vi "Periodic Tasks.vi"(8 "error in":errorcluster) -> ()   [LabVIEW 2013]
doc: "This VI runs in parallel to other tasks. It can contain as many user-defined periodic loops as you need. These can carry out PID or other sorts of timed response."
uses:
  <vilib>/Rock Robotics/WPI/DriverStation/DriverStationLCD/WPI_DriverStationLCDLCDLine.ctl
  <vilib>/Rock Robotics/SystemInterfaces/Utilities/FPGA_UtilitiesLED Source.ctl
  <vilib>/Rock Robotics/SystemInterfaces/Utilities/FPGA_UtilitiesLED State.ctl
  <vilib>/Rock Robotics/WPI/Relay/WPI_RelayValue.ctl
  <vilib>/Rock Robotics/WPI/SafetyOutput/WPI_SafetyOutputConfigMenu.ctl
  <vilib>/Rock Robotics/WPI/DriverStation/WPI_DriverStationRobotMode2.ctl
  <vilib>/Rock Robotics/WPI/Solenoid/WPI_SolenoidValue.ctl
  Begin/Global Refnums.vi
  <vilib>/Rock Robotics/WPI/Solenoid/WPI_SolenoidSetEnum.vi
  Begin/Robot Global Data.vi
  Begin/Global Variables.vi
  <vilib>/Rock Robotics/WPI/Joystick/WPI_JoystickGetSetRefNum.vi
  <vilib>/Rock Robotics/WPI/Compressor/WPI_CompressorGetSetRefNum.vi
panel:
  out "Fire":bool
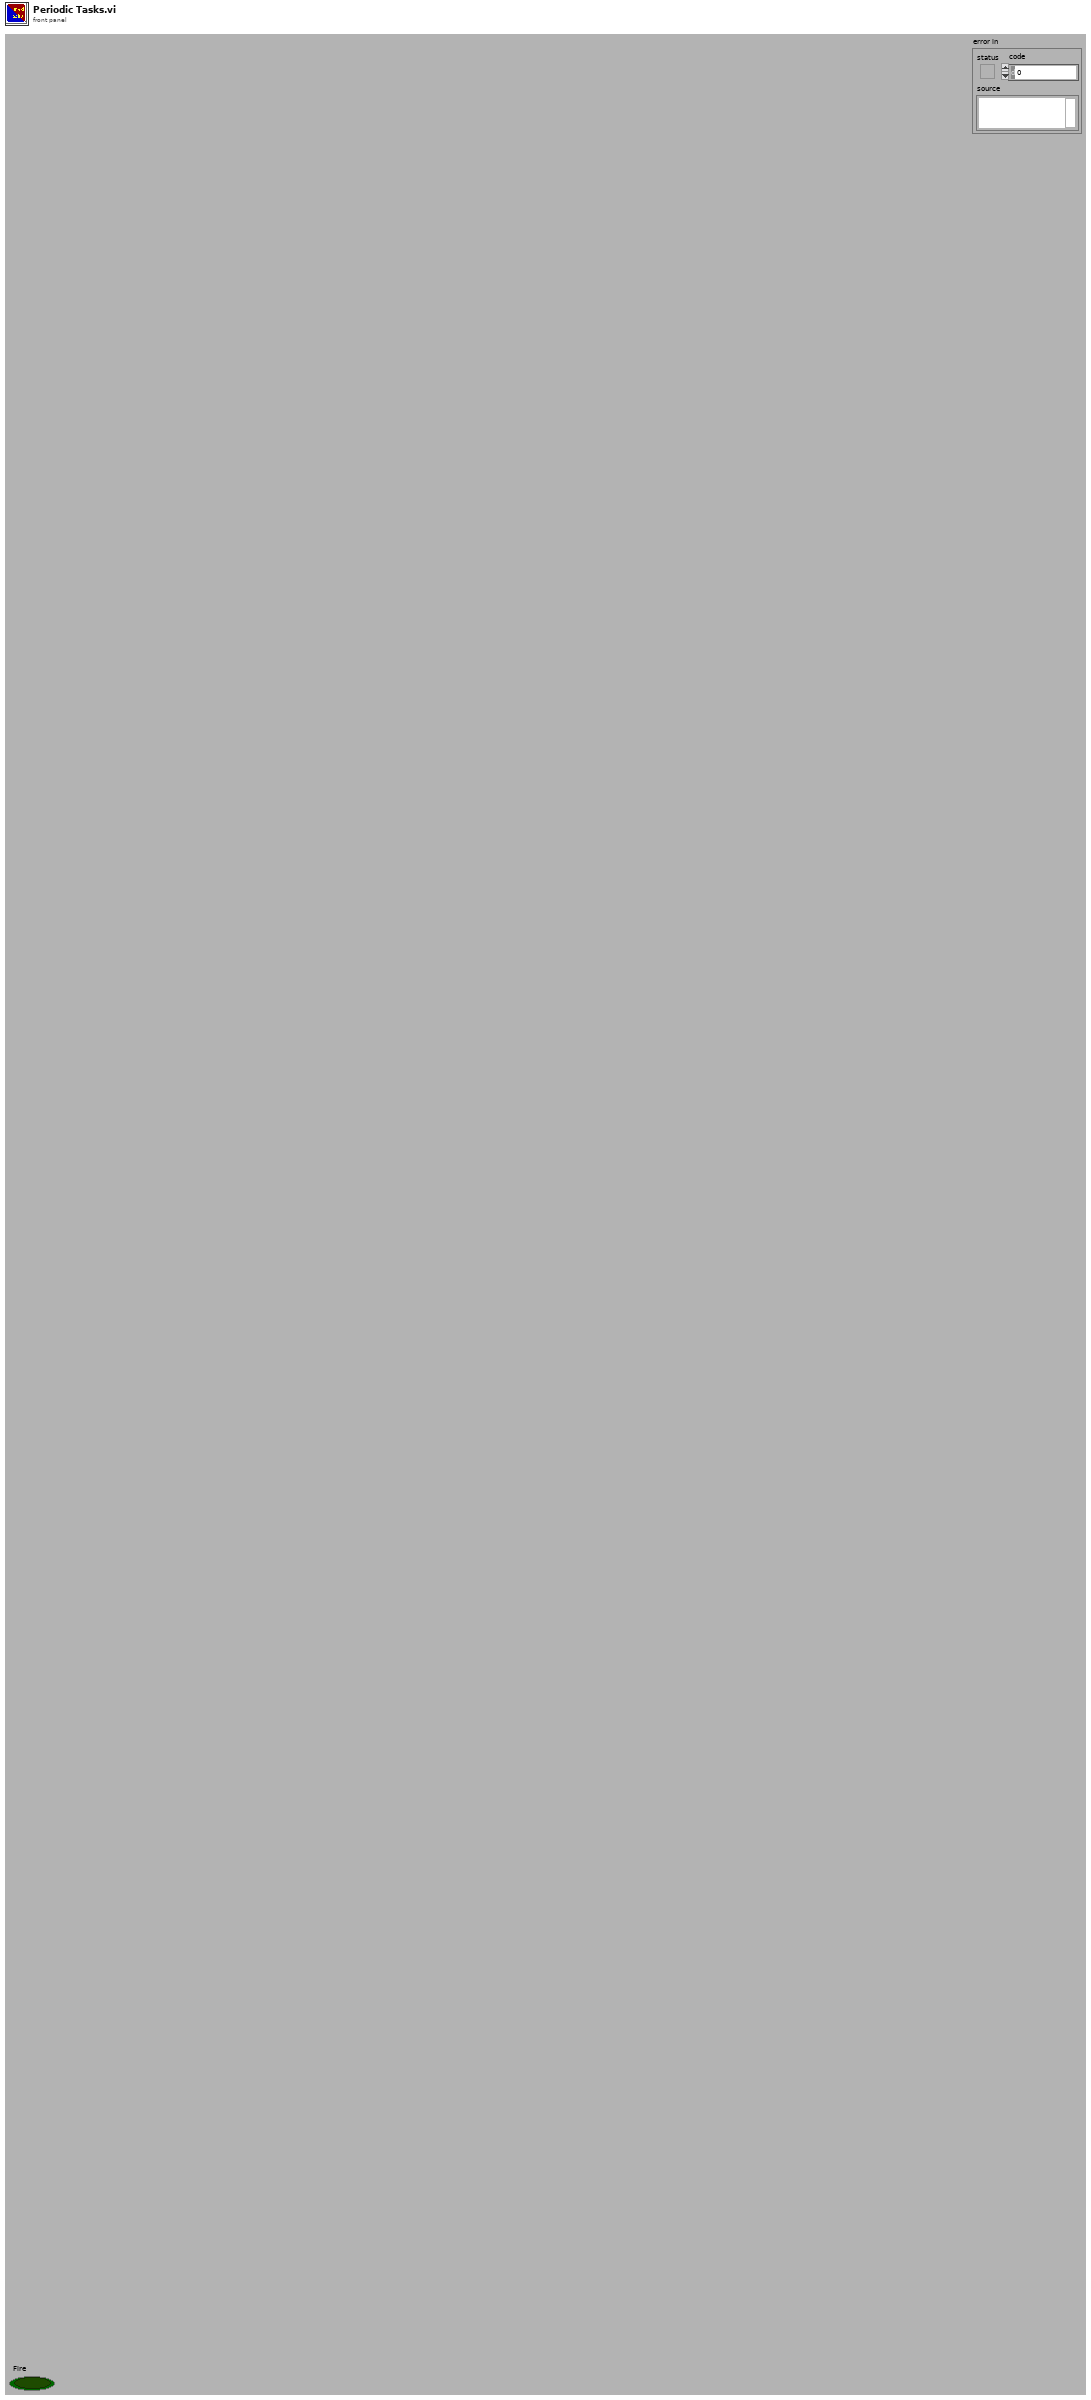
[diagram p1: front panel]
types:
  T1 = typedef "WPI_DriverStationLCDLCDLine.ctl" = enum16{"Main - Line 1", "User - Line 2", "User - Line 3", "User - Line 4", "User - Line 5", "User - Line 6"}
  T2 = typedef "WPI_SolenoidValue.ctl" = enum16{"Off", "On", "Forward", "Reverse"}
  T3 = typedef "WPI_SafetyOutputConfigMenu.ctl" = enum16{"Enable", "Disable"}
  T4 = typedef "WPI_SolenoidDevRef.ctl" = cluster{"DevStatus":errorcluster, "Solenoid Module":T5, "Forward Solenoid Channel":T6, "Reverse Solenoid Channel":T6}
  T5 = typedef "FPGA_TypedefSolenoidModule.ctl" = enum16{"Solenoid Module 1", "Solenoid Module 2"}
  T6 = typedef "WPI_SolenoidChannel.ctl" = enum8{"Solenoid 1", "Solenoid 2", "Solenoid 3", "Solenoid 4", "Solenoid 5", "Solenoid 6", "Solenoid 7", "Solenoid 8", "Invalid"}
  T7 = typedef "WPI_RelayValue.ctl" = enum16{"Off", "On", "Forward", "Reverse"}
  T8 = typedef "WPI_CompressorDevRef.ctl" = cluster{"DevStatus":errorcluster, "DigitalInputDevRef":T9, "RelayDevRef":T12}
  T9 = typedef "WPI_DigitalInputDevRef.ctl" = cluster{"DevStatus":errorcluster, "DIO Channel":T10, "Digital Module":T11}
  T10 = typedef "FPGA_DIOChannel.ctl" = enum8{"DIO 1", "DIO 2", "DIO 3", "DIO 4", "DIO 5", "DIO 6", "DIO 7", "DIO 8", "DIO 9", "DIO 10", "DIO 11", "DIO 12", "DIO 13", "DIO 14", "Invalid"}
  T11 = typedef "FPGA_TypedefDigitalModule.ctl" = enum16{"Digital Module 1", "Digital Module 2"}
  T12 = typedef "WPI_RelayDevRef.ctl" = cluster{"DevStatus":errorcluster, "Relay Channel":T13, "Digital Module":T11, "Relay Direction":T14}
  T13 = typedef "FPGA_DIORelayChannel.ctl" = enum8{"Relay 1", "Relay 2", "Relay 3", "Relay 4", "Relay 5", "Relay 6", "Relay 7", "Relay 8", "Invalid"}
  T14 = typedef "WPI_RelayDirection.ctl" = enum16{"Both directions", "Forward only", "Reverse only"}
  T15 = typedef "WPI_EncoderDevRef.ctl" = cluster{"DevStatus":errorcluster, "EncoderIndex":T16, "CounterIndex":T17, "DistancePerCount":dbl, "Decoding Type":T18}
  T16 = typedef "FPGA_EncoderIdx.ctl" = enum8{"Enc 0", "Enc 1", "Enc 2", "Enc 3", "Invalid"}
  T17 = typedef "FPGA_CounterCtrSystemIndex.ctl" = enum8{"Ctr 0", "Ctr 1", "Ctr 2", "Ctr 3", "Ctr 4", "Ctr 5", "Ctr 6", "Ctr 7", "Invalid"}
  T18 = typedef "WPI_EncoderType.ctl" = enum16{"1x", "2x", "4x"}
  T19 = typedef "WPI_DriverStationRobotMode2.ctl" = enum16{"Autonomous Disabled", "Autonomous Enabled", "Teleop Disabled", "Teleop Enabled", "Timeout", "Finish", "Test Disabled", "Test Enabled"}
  T20 = typedef "WPI_JoystickDevRef.ctl" = cluster{"Device":T21}
  T21 = typedef "WPI_JoystickDeviceEnum.ctl" = enum16{"USB 1", "USB 2", "USB 3", "USB 4", "Kinect 1", "Kinect 2"}
  T22 = typedef "WPI_JoystickButtonState.ctl" = cluster{"Button 1":bool, "Button 2":bool, "Button 3":bool, "Button 4":bool, "Button 5":bool, "Button 6":bool, "Button 7":bool, "Button 8":bool, "Button 9":bool, "Button 10":bool, "Button 11":bool, "Button 12":bool}
  T23 = typedef "WPI_MotorControlDeviceRef.ctl" = cluster{"DeviceStatus":errorcluster, "Type":enum16{"PWM", "CAN"}, "PWM":cluster{"Digital Module":T11, "PWM Channel":T24, "DeadBand":T25}, "CAN":cluster{"Device Number":u8, "Control Mode":T26, "Semaphore":T27, "Max Vout":dbl}, "Invert":bool, "TransformRef":T28, "InvTransformRef":T28}
  T24 = typedef "FPGA_DIOPWMChannel.ctl" = enum8{"PWM 1", "PWM 2", "PWM 3", "PWM 4", "PWM 5", "PWM 6", "PWM 7", "PWM 8", "PWM 9", "PWM 10", "Invalid"}
  T25 = typedef "WPI_PWMDeadband.ctl" = cluster{"Name":string, "maxPositivePwm":i32, "minPositivePwm":i32, "centerPwm":i32, "maxNegativePwm":i32, "minNegativePwm":i32, "angularRange":u16}
  T26 = typedef "WPI_CANJaguar_ControlMode.ctl" = enum8{"Percent VBus", "Current", "Speed", "Position", "Voltage"}
  T27 = typedef "Semaphore RefNum" = refnum<k1>
  T28 = typedef "WPI_PWMTransform_ConPane.ctl" = refnum<vi>
  T29 = typedef "FPGA_UtilitiesLED State.ctl" = enum16{"Off", "On", "Toggle"}
  T30 = typedef "FPGA_UtilitiesLED Source.ctl" = enum16{"User LED", "FPGA LED"}
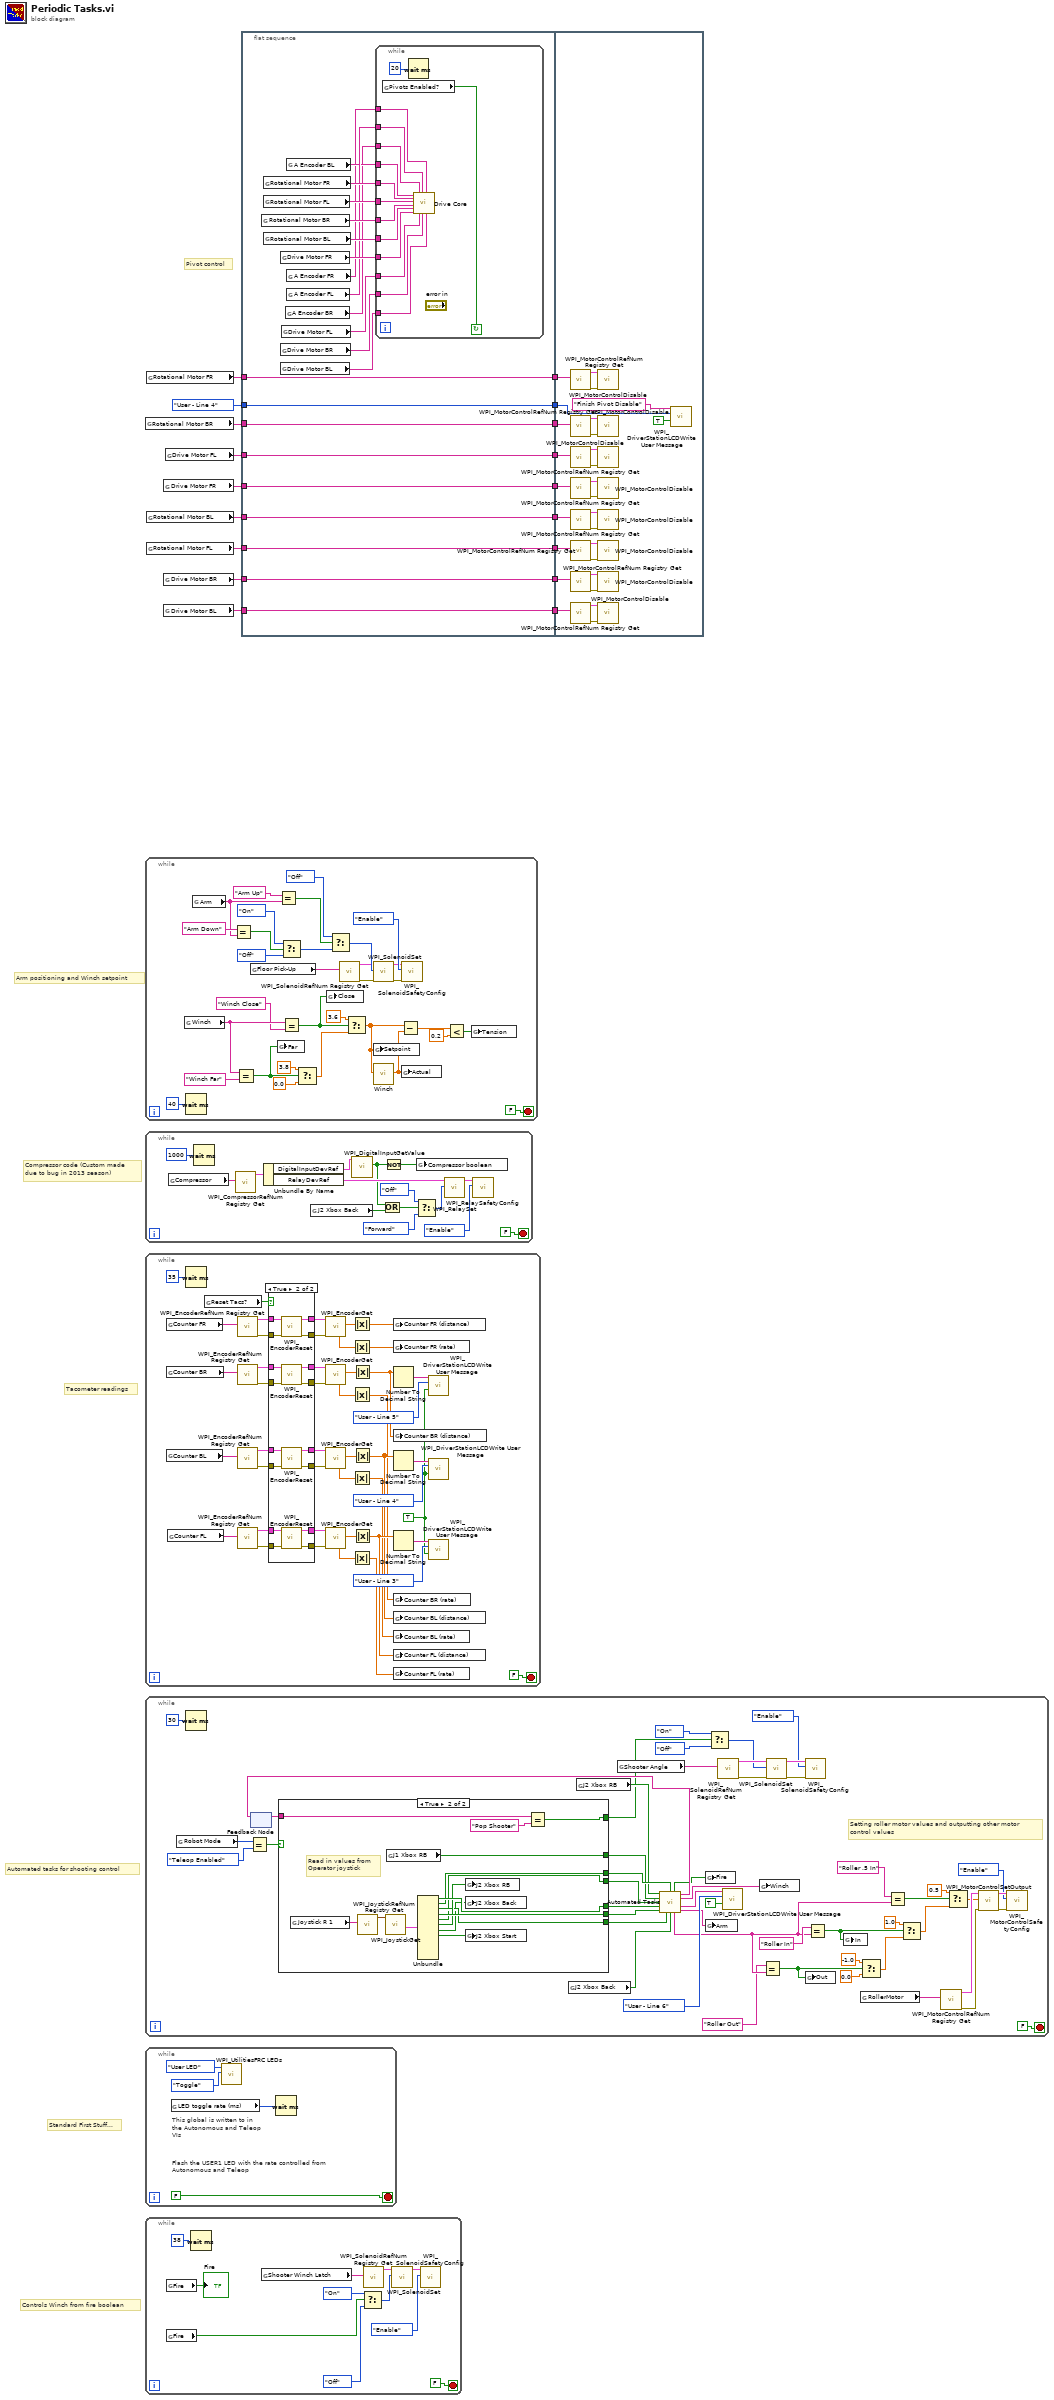
[diagram p0: block diagram]
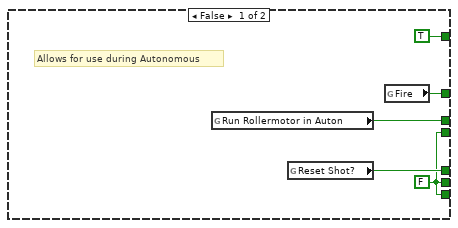
[diagram p2: hidden frame]
diagram:
  # "Automated tasks for shooting control"
  # "Tacometer readings"
  # "Compressor code (Custom made\ndue to bug in 2013 season)"
  # "Arm positioning and Winch setpoint"
  # "Pivot control"
  # "Standard First Stuff..."
  # "Controls Winch from fire boolean"
  n1 = global read "Global Refnums.vi" "Rotational Motor BR"() -> (w16:string)
  n2 = while {
    stop <- FALSE stop-if-true
    n3 = global read "Global Refnums.vi" "Winch"() -> (w50:string)
    n4 = Wait (ms)(milliseconds to wait=u32 40) -> ()  [unwired: 1 out]
    n5 = global read "Global Refnums.vi" "Arm"() -> (w24:string)
    n6 = Equal?(x="Arm Down", y=w24) -> (x = y?=w28:bool)
    n7 = Equal?(x=w50, y="Winch Far") -> (x = y?=w21:bool)
    n8 = global read "Global Refnums.vi" "Floor Pick-Up"() -> (w39:string)
    n9 = global write "Global Refnums.vi" "Far"(w21) -> ()
    n10 = Equal?(x="Arm Up", y=w24) -> (x = y?=w41:bool)
    n11 = Select(t=WPI_SolenoidValue."On" ("Value"), s=w28, f=WPI_SolenoidValue."Off" ("Value")) -> (s? t:f=w27:T2)
    n12 = Equal?(x=w50, y="Winch Close") -> (x = y?=w20:bool)
    n13 = Select(t=3.8, s=w21, f=0.0) -> (s? t:f=w47:dbl)
    n14 = global write "Global Refnums.vi" "Close"(w20) -> ()
    n15 = Select(t=WPI_SolenoidValue."Off" ("Value"), s=w41, f=w27) -> (s? t:f=w43:T2)
    n16 = call <vilib>:"WPI_SolenoidRefNum Registry Get.vi"("refnum name"=w39) -> ("error out"=w34:errorcluster, "SolenoidDevRef"=w35:T4)  [unwired: 9 in]
    n17 = Select(t=3.6, s=w20, f=w47) -> (s? t:f=w19:dbl)
    n18 = call-poly <vilib>:"WPI_SolenoidSet.vi"("error in (no error)"=w34, "Value"=w43, "SolenoidDevRef"=w35) -> ("error out"=w37:errorcluster, "SolenoidDevRef"=w36:T4)  [unwired: 7 in]
    n19 = global write "Global Refnums.vi" "Setpoint"(w19) -> ()
    n20 = call "Winch.vi"("setpoint"=w19) -> ("Actual"=w22:dbl)  [unwired: 10 in]
    n21 = Subtract(x=w19, y=w22) -> (x-y=w31:dbl)
    n22 = call <vilib>:"WPI_SolenoidSafetyConfig.vi"("error in (no error)"=w37, "mode"=WPI_SafetyOutputConfigMenu."Enable", "SolenoidDevRef"=w36) -> ()  [unwired: 7 in, 2 out]
    n23 = global write "Global Refnums.vi" "Actual"(w22) -> ()
    n24 = Less?(x=w31, y=0.2) -> (x < y?=w23:bool)
    n25 = global write "Global Refnums.vi" "Tension"(w23) -> ()
  }
  n26 = while {
    stop <- FALSE stop-if-true
    n27 = global read "Global Refnums.vi" "Compressor"() -> (w63:string)
    n28 = Wait (ms)(milliseconds to wait=1000) -> ()  [unwired: 1 out]
    n29 = call <vilib>:"WPI_CompressorRefNum Registry Get.vi"("refnum name"=w63) -> ("CompressorDevRef"=w62:T8)  [unwired: 9 in, 1 out]
    n30 = Unbundle By Name(w62) -> ("DigitalInputDevRef"=w55:T9, "RelayDevRef"=w61:T12)
    n31 = global read "Global Variables.vi" "J2 Xbox Back"() -> (w53:bool)
    n32 = call <vilib>:"WPI_DigitalInputGetValue.vi"("DigitalInputDevRef"=w55) -> ("Value"=w52:bool)  [unwired: 8 in, 2 out]
    n33 = Or(x=w52, y=w53) -> (x .or. y?=w54:bool)
    n34 = Not(x=w52) -> (.not. x?=w51:bool)
    n35 = Select(t=WPI_RelayValue."Off" ("RelayValue"), s=w54, f=WPI_RelayValue."Forward" ("RelayValue")) -> (s? t:f=w58:T7)
    n36 = global write "Global Refnums.vi" "Compressor boolean"(w51) -> ()
    n37 = call <vilib>:"WPI_RelaySet.vi"("RelayValue"=w58, "RelayDevRef"=w61) -> ("RelayDevRef"=w60:T12)  [unwired: 8 in, 1 out]
    n38 = call <vilib>:"WPI_RelaySafetyConfig.vi"("mode"=WPI_SafetyOutputConfigMenu."Enable", "RelayDevRef"=w60) -> ()  [unwired: 8 in, 2 out]
  }
  n39 = while {
    stop <- FALSE stop-if-true
    w67 = TRUE ("clear line before write (T)")
    n40 = global read "Global Refnums.vi" "Counter FR"() -> (w78:string)
    n41 = global read "Global Refnums.vi" "Counter BR"() -> (w76:string)
    n42 = global read "Global Refnums.vi" "Counter BL"() -> (w79:string)
    n43 = global read "Global Refnums.vi" "Counter FL"() -> (w77:string)
    n44 = Wait (ms)(milliseconds to wait=u32 35) -> ()  [unwired: 1 out]
    n45 = global read "Global Variables.vi" "Reset Tacs?"() -> (w66:bool)
    n46 = call <vilib>:"WPI_EncoderRefNum Registry Get.vi"("refnum name"=w78) -> ("error out"=w94:errorcluster, "EncoderDevRef"=w97:T15)  [unwired: 9 in]
    n47 = call <vilib>:"WPI_EncoderRefNum Registry Get.vi"("refnum name"=w76) -> ("error out"=w102:errorcluster, "EncoderDevRef"=w103:T15)  [unwired: 9 in]
    n48 = call <vilib>:"WPI_EncoderRefNum Registry Get.vi"("refnum name"=w79) -> ("error out"=w104:errorcluster, "EncoderDevRef"=w105:T15)  [unwired: 9 in]
    n49 = call <vilib>:"WPI_EncoderRefNum Registry Get.vi"("refnum name"=w77) -> ("error out"=w99:errorcluster, "EncoderDevRef"=w100:T15)  [unwired: 9 in]
    n50 = case shown="True" w66 {
      tunnel: w103 -> [w116 w135]
      tunnel: [w116 w134] -> w108
      tunnel: [w118 w133] -> w109
      tunnel: w102 -> [w118 w132]
      tunnel: [w117 w131] -> w107
      tunnel: [w119 w130] -> w106
      tunnel: w105 -> [w117 w129]
      tunnel: w104 -> [w119 w128]
      tunnel: [w115 w120] -> w101
      tunnel: w100 -> [w115 w127]
      tunnel: w99 -> [w114 w126]
      tunnel: [w114 w121] -> w98
      tunnel: w97 -> [w113 w125]
      tunnel: [w113 w122] -> w96
      tunnel: [w112 w123] -> w95
      tunnel: w94 -> [w112 w124]
      frame False {
      }
      frame True {
        n51 = call <vilib>:"WPI_EncoderReset.vi"("error in (no error)"=w124, "EncoderDevRef"=w125) -> ("error out"=w123:errorcluster, "EncoderDevRef"=w122:T15)  [unwired: 8 in]
        n52 = call <vilib>:"WPI_EncoderReset.vi"("error in (no error)"=w132, "EncoderDevRef"=w135) -> ("error out"=w133:errorcluster, "EncoderDevRef"=w134:T15)  [unwired: 8 in]
        n53 = call <vilib>:"WPI_EncoderReset.vi"("error in (no error)"=w128, "EncoderDevRef"=w129) -> ("error out"=w130:errorcluster, "EncoderDevRef"=w131:T15)  [unwired: 8 in]
        n54 = call <vilib>:"WPI_EncoderReset.vi"("error in (no error)"=w126, "EncoderDevRef"=w127) -> ("error out"=w121:errorcluster, "EncoderDevRef"=w120:T15)  [unwired: 8 in]
      }
    }
    n55 = call <vilib>:"WPI_EncoderGet.vi"("error in (no error)"=w95, "EncoderDevRef"=w96) -> ("Distance"=w91:dbl, "Rate"=w87:dbl)  [unwired: 4 in, 4 out]
    n56 = call <vilib>:"WPI_EncoderGet.vi"("error in (no error)"=w109, "EncoderDevRef"=w108) -> ("Distance"=w90:dbl, "Rate"=w86:dbl)  [unwired: 4 in, 4 out]
    n57 = call <vilib>:"WPI_EncoderGet.vi"("error in (no error)"=w106, "EncoderDevRef"=w107) -> ("Distance"=w92:dbl, "Rate"=w88:dbl)  [unwired: 4 in, 4 out]
    n58 = call <vilib>:"WPI_EncoderGet.vi"("error in (no error)"=w98, "EncoderDevRef"=w101) -> ("Distance"=w93:dbl, "Rate"=w89:dbl)  [unwired: 4 in, 4 out]
    n59 = Absolute Value(x=w91) -> (abs(x)=w75:dbl)
    n60 = Absolute Value(x=w87) -> (abs(x)=w74:dbl)
    n61 = Absolute Value(x=w86) -> (abs(x)=w68:dbl)
    n62 = Absolute Value(x=w88) -> (abs(x)=w70:dbl)
    n63 = Absolute Value(x=w89) -> (abs(x)=w72:dbl)
    n64 = Absolute Value(x=w90) -> (abs(x)=w69:dbl)
    n65 = Absolute Value(x=w92) -> (abs(x)=w71:dbl)
    n66 = Absolute Value(x=w93) -> (abs(x)=w73:dbl)
    n67 = global write "Global Refnums.vi" "Counter FR (distance)"(w75) -> ()
    n68 = global write "Global Refnums.vi" "Counter FR (rate)"(w74) -> ()
    n69 = Number To Decimal String(number=w69) -> (decimal integer string=w85:string)  [unwired: 1 in]
    n70 = global write "Global Refnums.vi" "Counter BR (distance)"(w69) -> ()
    n71 = Number To Decimal String(number=w71) -> (decimal integer string=w83:string)  [unwired: 1 in]
    n72 = Number To Decimal String(number=w73) -> (decimal integer string=w84:string)  [unwired: 1 in]
    n73 = global write "Global Refnums.vi" "Counter BR (rate)"(w68) -> ()
    n74 = global write "Global Refnums.vi" "Counter BL (distance)"(w71) -> ()
    n75 = global write "Global Refnums.vi" "Counter BL (rate)"(w70) -> ()
    n76 = global write "Global Refnums.vi" "Counter FL (distance)"(w73) -> ()
    n77 = global write "Global Refnums.vi" "Counter FL (rate)"(w72) -> ()
    n78 = call <vilib>:"WPI_DriverStationLCDWrite User Message.vi"("line text"=w85, "line"=WPI_DriverStationLCDLCDLine."User - Line 5", "clear line before write (T)"=w67) -> ()  [unwired: 12 in, 1 out]
    n79 = call <vilib>:"WPI_DriverStationLCDWrite User Message.vi"("line text"=w83, "line"=WPI_DriverStationLCDLCDLine."User - Line 4", "clear line before write (T)"=w67) -> ()  [unwired: 12 in, 1 out]
    n80 = call <vilib>:"WPI_DriverStationLCDWrite User Message.vi"("line text"=w84, "line"=WPI_DriverStationLCDLCDLine."User - Line 3", "clear line before write (T)"=w67) -> ()  [unwired: 12 in, 1 out]
  }
  n81 = while {
    stop <- FALSE stop-if-true
    # "Setting roller motor values and outputting other motor\ncontrol values"
    n82 = global read "Robot Global Data.vi" "Robot Mode"() -> (w157:T19)
    n83 = Wait (ms)(milliseconds to wait=u32 30) -> ()  [unwired: 1 out]
    n84 = Equal?(x=w157, y=WPI_DriverStationRobotMode2."Teleop Enabled") -> (x = y?=w158:bool)
    n85 = feedback #1() -> (w153:string)  [unwired: 1 in]
    n86 = case shown="True" w158 {
      tunnel: [w188 w203] -> w141
      tunnel: [w190 w202] -> w169
      tunnel: [w187 w201] -> w168
      tunnel: [w191 w200] -> w167
      tunnel: w153 -> [_ w198]
      tunnel: [TRUE w197] -> w152
      tunnel: [w187 w195] -> w150
      tunnel: [w187 w194] -> w142
      frame False {
        w187 = FALSE ("J1 Xbox RB")
        # "Allows for use during Autonomous"
        n87 = global read "Global Refnums.vi" "Run Rollermotor in Auton"() -> (w190:bool)
        n88 = global read "Global Refnums.vi" "Reset Shot?"() -> (w188:bool)
        n89 = global read "Global Refnums.vi" "Fire"() -> (w191:bool)
      }
      frame True {
        # "Read in values from \nOperator joystick"
        n90 = global read "Global Refnums.vi" "Joystick R 1"() -> (w204:string)
        n91 = call <vilib>:"WPI_JoystickRefNum Registry Get.vi"("refnum name"=w204) -> ("JoystickDevRef"=w206:T20)  [unwired: 9 in, 1 out]
        n92 = call <vilib>:"WPI_JoystickGet.vi"("JoystickDevRef"=w206) -> ("Buttons"=w205:T22)  [unwired: 4 in, 2 out]
        n93 = global read "Global Variables.vi" "J1 Xbox RB"() -> (w200:bool)
        n94 = Unbundle(w205) -> ("Button 1"=w203:bool, "Button 2"=w202:bool, "Button 3"=w195:bool, "Button 4"=w201:bool, "Button 5"=w194:bool, "Button 6"=w196:bool, "Button 7"=w193:bool, "Button 8"=w192:bool)  [unwired: 4 out]
        n95 = global write "Global Variables.vi" "J2 Xbox RB"(w196) -> ()
        n96 = global write "Global Variables.vi" "J2 Xbox Back"(w193) -> ()
        n97 = global write "Global Variables.vi" "J2 Xbox Start"(w192) -> ()
        n98 = Equal?(x=w198, y="Pop Shooter") -> (x = y?=w197:bool)
      }
    }
    n99 = global read "Global Variables.vi" "J2 Xbox Back"() -> (w138:bool)
    n100 = global read "Global Variables.vi" "J2 Xbox RB"() -> (w155:bool)
    n101 = global read "Global Refnums.vi" "Shooter Angle"() -> (w165:string)
    n102 = call "Automated Tasks.vi"("RB"=w155, "B"=w169, "Fire"=w167, "LB"=w142, "A"=w141, "Y"=w168, "X"=w150, "Back"=w138) -> ("Fire"=w151:bool, "Shooter"=w154:string, "Winch"=w140:string, "Case"=w163:string, "Roller"=w147:string, "Arm"=w160:string)  [unwired: 2 in]
    n103 = feedback-in #1(w154) -> ()
    n104 = global write "Global Refnums.vi" "Fire"(w151) -> ()
    n105 = global write "Global Refnums.vi" "Arm"(w160) -> ()
    n106 = Select(t=WPI_SolenoidValue."On" ("Value"), s=w152, f=WPI_SolenoidValue."Off" ("Value")) -> (s? t:f=w170:T2)
    n107 = call <vilib>:"WPI_SolenoidRefNum Registry Get.vi"("refnum name"=w165) -> ("error out"=w177:errorcluster, "SolenoidDevRef"=w176:T4)  [unwired: 9 in]
    n108 = call <vilib>:"WPI_DriverStationLCDWrite User Message.vi"("line text"=w163, "line"=WPI_DriverStationLCDLCDLine."User - Line 6", "clear line before write (T)"=TRUE) -> ()  [unwired: 12 in, 1 out]
    n109 = global write "Global Refnums.vi" "Winch"(w140) -> ()
    n110 = Equal?(x="Roller Out", y=w147) -> (x = y?=w136:bool)
    n111 = call-poly <vilib>:"WPI_SolenoidSet.vi"("error in (no error)"=w177, "Value"=w170, "SolenoidDevRef"=w176) -> ("error out"=w174:errorcluster, "SolenoidDevRef"=w175:T4)  [unwired: 7 in]
    n112 = call <vilib>:"WPI_SolenoidSafetyConfig.vi"("error in (no error)"=w174, "mode"=WPI_SafetyOutputConfigMenu."Enable", "SolenoidDevRef"=w175) -> ()  [unwired: 7 in, 2 out]
    n113 = global write "Global Refnums.vi" "Out"(w136) -> ()
    n114 = Equal?(x="Roller In", y=w147) -> (x = y?=w137:bool)
    n115 = global write "Global Refnums.vi" "In"(w137) -> ()
    n116 = Select(t=-1.0, s=w136, f=0.0) -> (s? t:f=w178:dbl)
    n117 = global read "Global Refnums.vi" "RollerMotor"() -> (w166:string)
    n118 = Equal?(x="Roller .5 In", y=w147) -> (x = y?=w146:bool)
    n119 = Select(t=1.0, s=w137, f=w178) -> (s? t:f=w145:dbl)
    n120 = call <vilib>:"WPI_MotorControlRefNum Registry Get.vi"("refnum name"=w166) -> ("error out"=w184:errorcluster, "MotorControlDevRef"=w186:T23)  [unwired: 9 in]
    n121 = Select(t=0.5, s=w146, f=w145) -> (s? t:f=w149:dbl)
    n122 = call <vilib>:"WPI_MotorControlSetOutput.vi"("error in (no error)"=w184, "Output"=w149, "MotorControlDevRef"=w186) -> ("error out"=w183:errorcluster, "MotorControlDevRef"=w185:T23)  [unwired: 6 in, 1 out]
    n123 = call <vilib>:"WPI_MotorControlSafetyConfig.vi"("error in (no error)"=w183, "mode"=WPI_SafetyOutputConfigMenu."Enable", "MotorControlDevRef"=w185) -> ()  [unwired: 7 in, 2 out]
  }
  n124 = while {
    stop <- FALSE stop-if-true
    # "This global is written to in the Autonomous and Teleop VIs"
    # "Flash the USER1 LED with the rate controlled from Autonomous and Teleop"
    n125 = global read "Robot Global Data.vi" "LED toggle rate (ms)"() -> (w207:u32)
    n126 = call <vilib>:"WPI_UtilitiesFRC LEDs.vi"("State"=FPGA_UtilitiesLED_State."Toggle", "LED Type"=FPGA_UtilitiesLED_Source."User LED") -> ()  [unwired: 1 in, 9 out]
    n127 = Wait (ms)(milliseconds to wait=w207) -> ()  [unwired: 1 out]
  }
  n128 = while {
    stop <- FALSE stop-if-true
    n129 = global read "Global Refnums.vi" "Fire"() -> (→"Fire":bool)
    n130 = global read "Global Refnums.vi" "Fire"() -> (w211:bool)
    n131 = Wait (ms)(milliseconds to wait=u32 38) -> ()  [unwired: 1 out]
    n132 = global read "Global Refnums.vi" "Shooter Winch Latch"() -> (w217:string)
    n133 = Select(t=WPI_SolenoidValue."On", s=w211, f=WPI_SolenoidValue."Off" ("Value")) -> (s? t:f=w212:T2)
    n134 = call <vilib>:"WPI_SolenoidRefNum Registry Get.vi"("refnum name"=w217) -> ("SolenoidDevRef"=w218:T4)  [unwired: 9 in, 1 out]
    n135 = call-poly <vilib>:"WPI_SolenoidSet.vi"("Value"=w212, "SolenoidDevRef"=w218) -> ("SolenoidDevRef"=w219:T4)  [unwired: 8 in, 1 out]
    n136 = call <vilib>:"WPI_SolenoidSafetyConfig.vi"("mode"=WPI_SafetyOutputConfigMenu."Enable", "SolenoidDevRef"=w219) -> ()  [unwired: 8 in, 2 out]
  }
  n137 = global read "Global Refnums.vi" "Rotational Motor FR"() -> (w18:string)
  n138 = global read "Global Refnums.vi" "Rotational Motor BL"() -> (w15:string)
  n139 = global read "Global Refnums.vi" "Rotational Motor FL"() -> (w17:string)
  n140 = global read "Global Refnums.vi" "Drive Motor FR"() -> (w14:string)
  n141 = global read "Global Refnums.vi" "Drive Motor BR"() -> (w12:string)
  n142 = global read "Global Refnums.vi" "Drive Motor BL"() -> (w11:string)
  n143 = global read "Global Refnums.vi" "Drive Motor FL"() -> (w13:string)
  n144 = flat-sequence {
    tunnel: WPI_DriverStationLCDLCDLine."User - Line 4" ("line") -> [w234]
    tunnel: w13 -> [w235]
    tunnel: w11 -> [w236]
    tunnel: w12 -> [w237]
    tunnel: w14 -> [w238]
    tunnel: w15 -> [w239]
    tunnel: w16 -> [w240]
    tunnel: w17 -> [w241]
    tunnel: w18 -> [w242]
    tunnel: [w242] -> w9
    tunnel: [w241] -> w8
    tunnel: [w240] -> w7
    tunnel: [w239] -> w6
    tunnel: [w238] -> w5
    tunnel: [w237] -> w4
    tunnel: [w236] -> w3
    tunnel: [w235] -> w2
    tunnel: [w234] -> w1
    tunnel: w9 -> [w283]
    tunnel: w8 -> [w276]
    tunnel: w7 -> [w275]
    tunnel: w6 -> [w272]
    tunnel: w5 -> [w263]
    tunnel: w4 -> [w262]
    tunnel: w3 -> [w261]
    tunnel: w2 -> [w260]
    tunnel: w1 -> [w259]
    frame #0 {
      n145 = global read "Global Refnums.vi" "Rotational Motor BR"() -> (w228:string)
      n146 = global read "Global Refnums.vi" "Rotational Motor FR"() -> (w226:string)
      n147 = global read "Global Refnums.vi" "Rotational Motor FL"() -> (w227:string)
      n148 = global read "Global Refnums.vi" "Rotational Motor BL"() -> (w229:string)
      n149 = global read "Global Refnums.vi" "Drive Motor FR"() -> (w230:string)
      n150 = global read "Global Refnums.vi" "Drive Motor BR"() -> (w232:string)
      n151 = global read "Global Refnums.vi" "Drive Motor BL"() -> (w233:string)
      n152 = global read "Global Refnums.vi" "Drive Motor FL"() -> (w231:string)
      n153 = global read "Global Refnums.vi" "A Encoder BR"() -> (w223:string)
      n154 = global read "Global Refnums.vi" "A Encoder BL"() -> (w224:string)
      n155 = global read "Global Refnums.vi" "A Encoder FR"() -> (w222:string)
      n156 = global read "Global Refnums.vi" "A Encoder FL"() -> (w225:string)
      n157 = while {
        tunnel: w222 -> [w256]
        tunnel: w223 -> [w254]
        tunnel: w224 -> [w253]
        tunnel: w225 -> [w255]
        tunnel: w230 -> [w248]
        tunnel: w232 -> [w246]
        tunnel: w233 -> [w245]
        tunnel: w231 -> [w247]
        tunnel: w226 -> [w252]
        tunnel: w228 -> [w250]
        tunnel: w229 -> [w249]
        tunnel: w227 -> [w251]
        stop <- w243 continue-if-true
        n158 = global read "Global Variables.vi" "Pivots Enabled?"() -> (w243:bool)
        n159 = Wait (ms)(milliseconds to wait=u32 20) -> ()  [unwired: 1 out]
        n160 = call "Drive Core.vi"("A Encoder BL"=w253, "Rotational Motor FR"=w252, "Rotational Motor FL"=w251, "Rotational Motor BR"=w250, "Rotational Motor BL"=w249, "Drive Motor FR"=w248, "A Encoder BR"=w254, "Drive Motor FL"=w247, "A Encoder FL"=w255, "Drive Motor BR"=w246, "A Encoder FR"=w256, "Drive Motor BL"=w245) -> ()  [unwired: 8 in]
      }
    }
    frame #1 {
      n161 = call <vilib>:"WPI_MotorControlRefNum Registry Get.vi"("refnum name"=w283) -> ("error out"=w281:errorcluster, "MotorControlDevRef"=w282:T23)  [unwired: 9 in]
      n162 = call <vilib>:"WPI_MotorControlRefNum Registry Get.vi"("refnum name"=w275) -> ("error out"=w277:errorcluster, "MotorControlDevRef"=w278:T23)  [unwired: 9 in]
      n163 = call <vilib>:"WPI_MotorControlRefNum Registry Get.vi"("refnum name"=w260) -> ("error out"=w267:errorcluster, "MotorControlDevRef"=w266:T23)  [unwired: 9 in]
      n164 = call <vilib>:"WPI_MotorControlRefNum Registry Get.vi"("refnum name"=w263) -> ("error out"=w265:errorcluster, "MotorControlDevRef"=w264:T23)  [unwired: 9 in]
      n165 = call <vilib>:"WPI_MotorControlRefNum Registry Get.vi"("refnum name"=w272) -> ("error out"=w273:errorcluster, "MotorControlDevRef"=w274:T23)  [unwired: 9 in]
      n166 = call <vilib>:"WPI_MotorControlRefNum Registry Get.vi"("refnum name"=w276) -> ("error out"=w279:errorcluster, "MotorControlDevRef"=w280:T23)  [unwired: 9 in]
      n167 = call <vilib>:"WPI_MotorControlRefNum Registry Get.vi"("refnum name"=w262) -> ("error out"=w269:errorcluster, "MotorControlDevRef"=w268:T23)  [unwired: 9 in]
      n168 = call <vilib>:"WPI_MotorControlRefNum Registry Get.vi"("refnum name"=w261) -> ("error out"=w271:errorcluster, "MotorControlDevRef"=w270:T23)  [unwired: 9 in]
      n169 = call <vilib>:"WPI_MotorControlDisable.vi"("error in (no error)"=w281, "MotorControlDevRef"=w282) -> ()  [unwired: 8 in, 2 out]
      n170 = call <vilib>:"WPI_MotorControlDisable.vi"("error in (no error)"=w277, "MotorControlDevRef"=w278) -> ()  [unwired: 8 in, 2 out]
      n171 = call <vilib>:"WPI_MotorControlDisable.vi"("error in (no error)"=w267, "MotorControlDevRef"=w266) -> ()  [unwired: 8 in, 2 out]
      n172 = call <vilib>:"WPI_MotorControlDisable.vi"("error in (no error)"=w265, "MotorControlDevRef"=w264) -> ()  [unwired: 8 in, 2 out]
      n173 = call <vilib>:"WPI_MotorControlDisable.vi"("error in (no error)"=w273, "MotorControlDevRef"=w274) -> ()  [unwired: 8 in, 2 out]
      n174 = call <vilib>:"WPI_MotorControlDisable.vi"("error in (no error)"=w279, "MotorControlDevRef"=w280) -> ()  [unwired: 8 in, 2 out]
      n175 = call <vilib>:"WPI_MotorControlDisable.vi"("error in (no error)"=w269, "MotorControlDevRef"=w268) -> ()  [unwired: 8 in, 2 out]
      n176 = call <vilib>:"WPI_MotorControlDisable.vi"("error in (no error)"=w271, "MotorControlDevRef"=w270) -> ()  [unwired: 8 in, 2 out]
      n177 = call <vilib>:"WPI_DriverStationLCDWrite User Message.vi"("line text"="Finish Pivot Disable", "line"=w259, "clear line before write (T)"=TRUE) -> ()  [unwired: 12 in, 1 out]
    }
  }
